vi "Main.vi"() -> ()   [LabVIEW 2015]
uses:
  TypeDefs/Queue Data.ctl
  SubVIs/App Data.vi
  SubVIs/App Strings.vi
  FGV/Timer Actions.ctl
  C:/Users/Student/Documents/209412/Lab7/Kody/Laboratorium 7/Finite Acquisition - Solution/FGV/Global 1.vi
panel:
  in  "Period [s]":dbl
  in  "Device name":tag="myDAQ1"
  out "Time Elapsed":dbl format="%<%M:%S>t"
  out "Status":string
  in  "Time [ms]":dbl
  in  "Frequency":dbl
  in  "Stop Button":bool
  in  "Acquire Button":bool
  out "Waveform Graph":dbl[](graph)
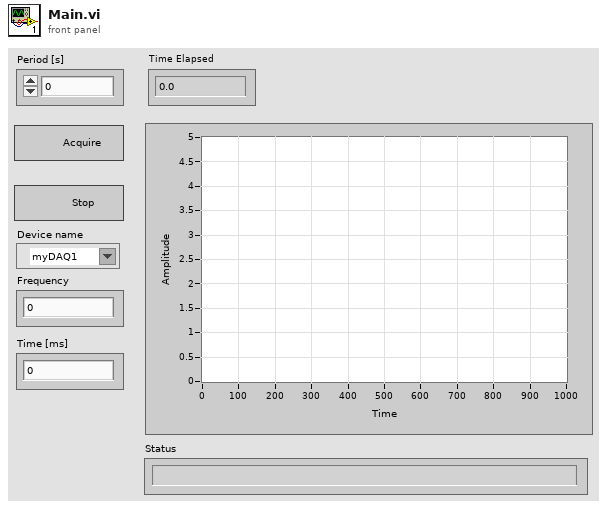
[diagram p1: front panel]
types:
  T1 = typedef "Timer Actions.ctl" = enum16{"Reset", "Get"}
  T2 = typedef "Queue Data.ctl" = cluster{"Action":string}
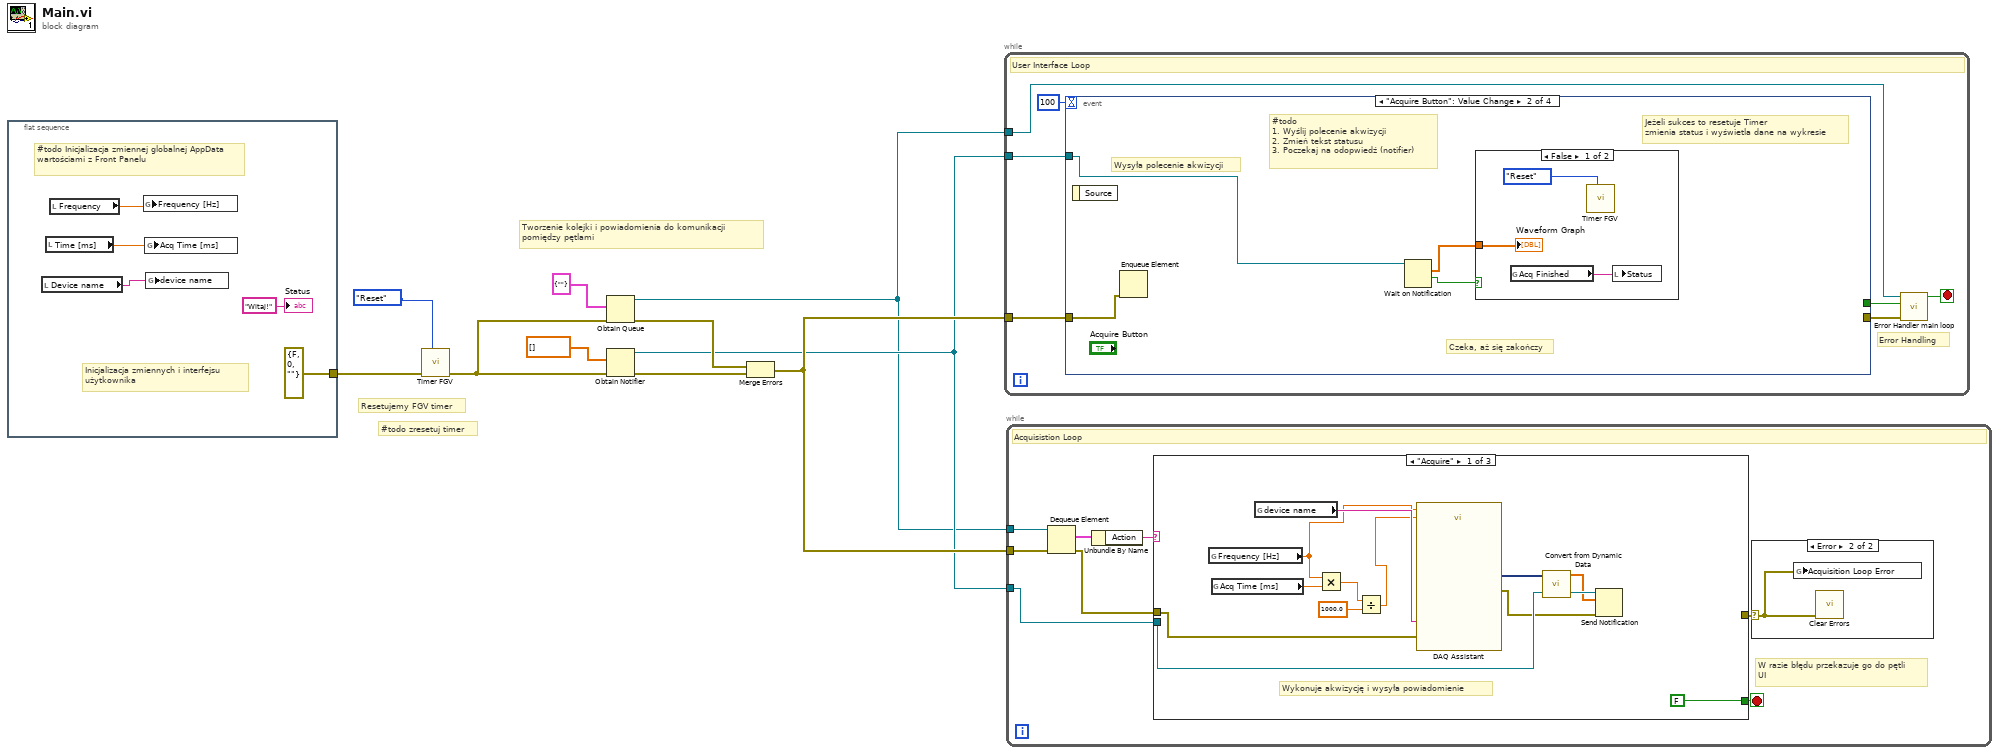
[diagram p0: block diagram]
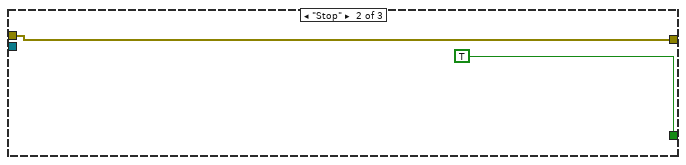
[diagram p3: hidden frame]
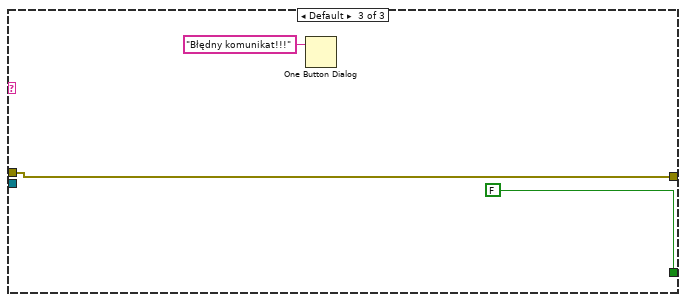
[diagram p4: hidden frame]
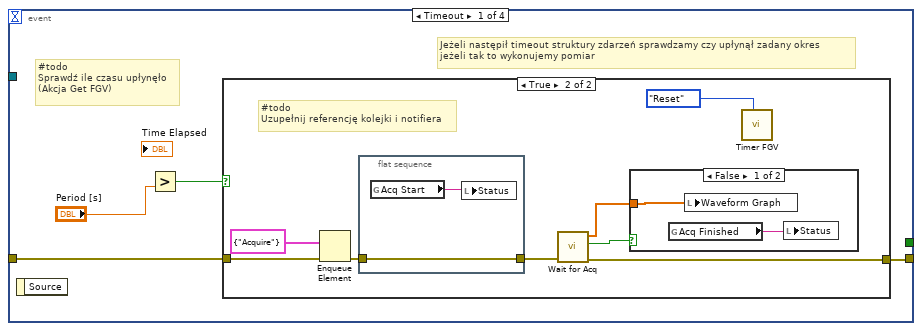
[diagram p5: hidden frame]
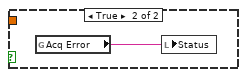
[diagram p7: hidden frame]
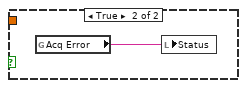
[diagram p8: hidden frame]
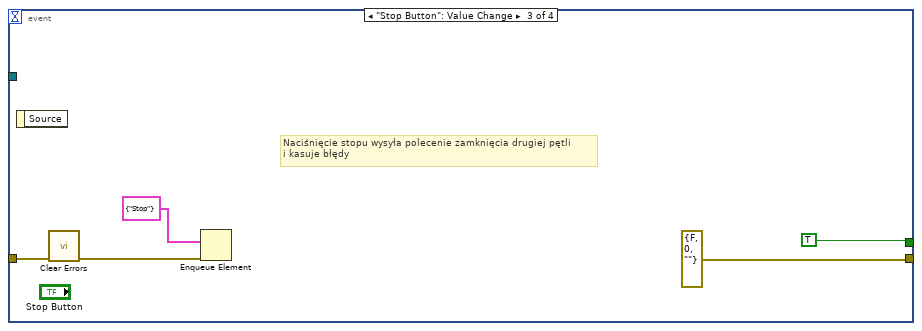
[diagram p9: hidden frame]
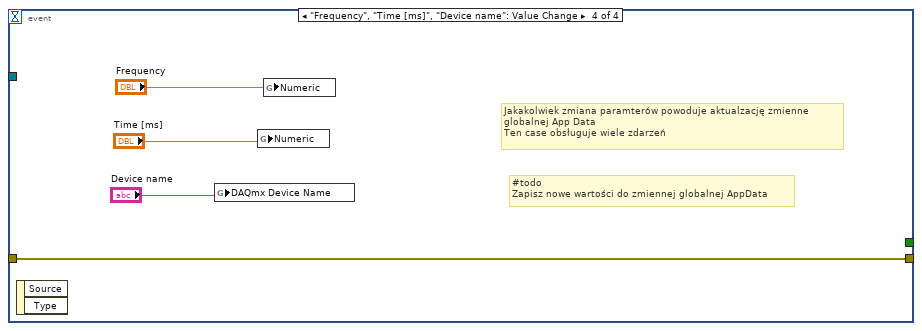
[diagram p10: hidden frame]
diagram:
  # "#todo zresetuj timer"
  # "Resetujemy FGV timer"
  # "Tworzenie kolejki i powiadomienia do komunikacji \npomiędzy pętlami"
  n1 = flat-sequence {
    tunnel: [errorcluster {"status"=FALSE, "code"=0, "source"=""} ("error constant")] -> w3
    frame #0 {
      # "#todo Inicjalizacja zmiennej globalnej AppData wartościami z Front Panelu"
      # "Inicjalizacja zmiennych i interfejsu \nużytkownika"
      n2 = local read "Device name"() -> (w11:tag)
      n3 = local read "Time [ms]"() -> (w12:dbl)
      n4 = local read "Frequency"() -> (w13:dbl)
      n5 = global write "App Data.vi" "Frequency [Hz]"(w13) -> ()
      n6 = global write "App Data.vi" "Acq Time [ms]"(w12) -> ()
      n7 = global write "App Data.vi" "device name"(w11) -> ()
      "Status" <- "Witaj!" ("Status")
    }
  }
  n8 = call "Timer FGV.vi"("Action"=Timer_Actions."Reset", "error in (no error)"=w3) -> ("error out"=w2:errorcluster)  [unwired: 8 in, 1 out]
  n9 = Obtain Queue(element data type=T2 {"Action"=""}, error in (no error)=w2) -> (queue out=w4:refnum<queue>, error out=w9:errorcluster)  [unwired: 3 in, 1 out]
  n10 = Obtain Notifier(notification data type=dbl[] [], error in (no error)=w2) -> (notifier out=w5:refnum<notifier>, error out=w7:errorcluster)  [unwired: 2 in, 1 out]
  n11 = Merge Errors(w9, w7) -> (w6:errorcluster)
  n12 = while {
    tunnel: w6 -> [w21]
    tunnel: w4 -> [w17]
    tunnel: w5 -> [w16]
    stop <- w18 stop-if-true
    # "Error Handling"
    # "User Interface Loop"
    n13 = event shown="[1] \"Acquire Button\": Value Change" {
      selector: _ -> [_ _ _ _]
      dyn-events: _ -> [_ _ _ _]
      timeout: 100 -> [_ _ _ _]
      tunnel: w21 -> [w24 w44 w50 w57]
      tunnel: [w23 _ errorcluster {"status"=FALSE, "code"=0, "source"=""} ("error constant") w57] -> w19
      tunnel: [_ _ TRUE _] -> w20
      tunnel: w16 -> [_ w43 _ _]
      event Timeout {
        # "#todo\nSprawdź ile czasu upłynęło\n(Akcja Get FGV)"
        # "Jeżeli następił timeout struktury zdarzeń sprawdzamy czy upłynął zadany okres \njeżeli tak to wykonujemy pomiar"
        n14 = event-data() -> ()  [unwired: 1 in, 1 out]
        n15 = Greater?(y="Period [s]") -> (0:w25:bool)  [unwired: 1 in]
        n16 = case shown="True" w25 {
          tunnel: w24 -> [w27 w35]
          tunnel: [w27 w28] -> w23
          frame False {
          }
          frame True {
            # "#todo\nUzupełnij referencję kolejki i notifiera"
            n17 = Enqueue Element(element=T2 {"Action"="Acquire"}, error in (no error)=w35) -> (error out=w33:errorcluster)  [unwired: 2 in, 2 out]
            n18 = flat-sequence {
              tunnel: w33 -> [w39]
              tunnel: [w39] -> w32
              frame #0 {
                n19 = global read "App Strings.vi" "Acq Start"() -> (w40:string)
                n20 = local write "Status"(w40) -> ()
              }
            }
            n21 = call "Wait for Acq.vi"("error in (no error)"=w32) -> ("error out"=w28:errorcluster, "timed out?"=w29:bool, "Array"=w31:dbl[])  [unwired: 8 in]
            n22 = case shown="False" w29 {
              tunnel: w31 -> [w36 _]
              frame False {
                n23 = global read "App Strings.vi" "Acq Finished"() -> (w37:string)
                n24 = local write "Waveform Graph"(w36) -> ()
                n25 = local write "Status"(w37) -> ()
              }
              frame True {
                n26 = global read "App Strings.vi" "Acq Error"() -> (w38:string)
                n27 = local write "Status"(w38) -> ()
              }
            }
            n28 = call "Timer FGV.vi"("Action"=Timer_Actions."Reset") -> ()  [unwired: 9 in, 2 out]
          }
        }
      }
      event "Acquire Button": Value Change {
        # "#todo\n1. Wyślij polecenie akwizycji\n2. Zmień tekst statusu\n3. Poczekaj na odopwiedź (notifier)"
        # "Jeżeli sukces to resetuje Timer\nzmienia status i wyświetla dane na wykresie"
        # "Czeka, aż się zakończy"
        # "Wysyła polecenie akwizycji"
        n29 = event-data() -> ()  [unwired: 1 in, 1 out]
        n30 = Enqueue Element(error in (no error)=w44) -> ()  [unwired: 3 in, 3 out]
        n31 = Wait on Notification(notifier=w43) -> (notification=w42:dbl[], timed out?=w41:bool)  [unwired: 3 in, 2 out]
        n32 = case shown="False" w41 {
          tunnel: w42 -> [w45 _]
          frame False {
            n33 = global read "App Strings.vi" "Acq Finished"() -> (w47:string)
            n34 = call "Timer FGV.vi"("Action"=Timer_Actions."Reset") -> ()  [unwired: 9 in, 2 out]
            n35 = local write "Status"(w47) -> ()
            "Waveform Graph" <- w45
          }
          frame True {
            n36 = global read "App Strings.vi" "Acq Error"() -> (w48:string)
            n37 = local write "Status"(w48) -> ()
          }
        }
      }
      event "Stop Button": Value Change {
        # "Naciśnięcie stopu wysyła polecenie zamknięcia drugiej pętli\ni kasuje błędy"
        n38 = event-data() -> ()  [unwired: 1 in, 1 out]
        n39 = call <vilib>:"Clear Errors.vi"("error in (no error)"=w50) -> ("error out"=w49:errorcluster)  [unwired: 5 in, 1 out]
        n40 = Enqueue Element(element=T2 {"Action"="Stop"}, error in (no error)=w49) -> ()  [unwired: 2 in, 3 out]
      }
      event "Frequency", "Time [ms]", "Device name": Value Change {
        # "#todo \nZapisz nowe wartości do zmiennej globalnej AppData"
        # "Jakakolwiek zmiana paramterów powoduje aktualzację zmienne \nglobalnej App Data\nTen case obsługuje wiele zdarzeń"
        n41 = event-data() -> ()  [unwired: 1 in, 2 out]
        n42 = global write "Global 1.vi" "DAQmx Device Name"("Device name") -> ()
        n43 = global write "Global 1.vi" "Numeric"("Time [ms]") -> ()
        n44 = global write "Global 1.vi" "Numeric"("Frequency") -> ()
      }
    }
    n45 = call "Error Handler main loop.vi"("error in (no error)"=w19, "Exit?"=w20, "Queue in"=w17) -> ("Exit?"=w18:bool)  [unwired: 8 in]
  }
  n46 = while {
    tunnel: w6 -> [w63]
    tunnel: w4 -> [w62]
    tunnel: w5 -> [w58]
    stop <- w60 stop-if-true
    # "W razie błędu przekazuje go do pętli\nUI"
    # "Acquisistion Loop"
    n47 = Dequeue Element(queue=w62, error in (no error)=w63) -> (element=w65:T2, error out=w61:errorcluster)  [unwired: 1 in, 2 out]
    n48 = Unbundle By Name(w65) -> ("Action"=w64:string)
    n49 = case shown="\"Acquire\"" w64 {
      tunnel: w61 -> [w74 w79 w82]
      tunnel: [FALSE TRUE FALSE] -> w60
      tunnel: [_ w79 w82] -> w59
      tunnel: w58 -> [w76 _ _]
      frame "Acquire" {
        # "Wykonuje akwizycję i wysyła powiadomienie"
        n50 = global read "App Data.vi" "Frequency [Hz]"() -> (w70:dbl)
        n51 = global read "App Data.vi" "Acq Time [ms]"() -> (w77:dbl)
        n52 = global read "App Data.vi" "device name"() -> (w75:tag)
        n53 = Multiply(x=w70, y=w77) -> (x*y=w69:dbl)
        n54 = Divide(x=w69, y=1000.0) -> (x/y=w68:dbl)
        n55 = call "DAQ Assistant"("rate"=w70, "number of samples"=w68, "error in"=w74, "device name"=w75) -> ("data"=w72:dynamicdata, "error out"=w73:errorcluster)  [unwired: 13 in, 1 out]
        n56 = call "Convert from Dynamic Data"("Dynamic Data Type"=w72) -> ("Array"=w71:dbl[])  [unwired: 3 in]
        n57 = Send Notification(notification=w71, notifier=w76, error in (no error)=w73) -> ()  [unwired: 2 out]
      }
      frame "Stop" {
      }
      frame Default {
        n58 = One Button Dialog(message="Błędny komunikat!!!") -> ()  [unwired: 1 in, 1 out]
      }
    }
    n59 = case shown="Error" w59 {
      selector: w59 -> [_ w66]
      frame No Error {
      }
      frame Error {
        n60 = global write "App Data.vi" "Acquisition Loop Error"(w66) -> ()
        n61 = call <vilib>:"Clear Errors.vi"("error in (no error)"=w66) -> ()  [unwired: 5 in, 2 out]
      }
    }
  }
